vi "Find Program Files.vi"() -> (2 "filenames":string[](array[string]), 3 "Array":string[](array[string]))   [LabVIEW 2025]
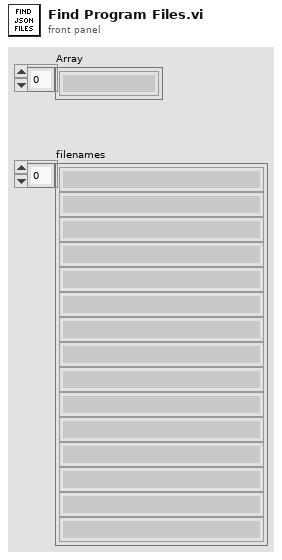
[diagram p1: front panel]
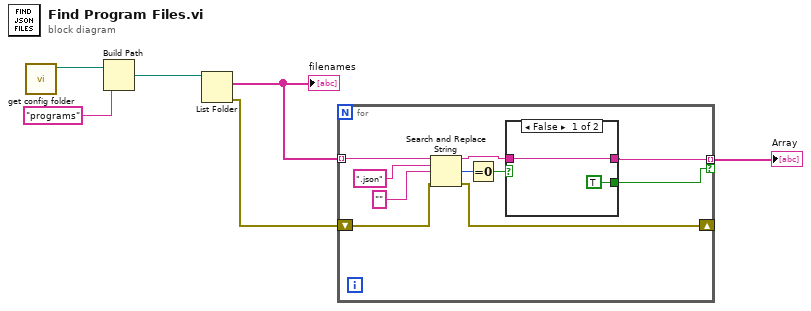
[diagram p0: block diagram]
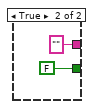
[diagram p2: hidden frame]
diagram:
  n1 = call "get config folder.vi"() -> ("Config folder path"=w1:path)  [unwired: 11 in]
  n2 = Build Path(base path=w1, name or relative path="programs") -> (appended path=w3:path)
  n3 = List Folder(path=w3) -> (filenames=w4:string[], error out=w5:errorcluster)  [unwired: 3 in, 2 out]
  "filenames" <- w4
  n4 = for {
    tunnel: w4 -> [w16] mode=indexing
    shift-right: [w11] -> _
    shift-left: w5 -> [w12]
    tunnel: [w8] -> w6 mode=indexing if=w7
    n5 = Search and Replace String(input string=w16, search string=".json", replace string="" ("replace string (\"\")"), error in=w12) -> (result string=w9:string, number of replacements=w14:i32, error out=w11:errorcluster)  [unwired: 4 in, 1 out]
    n6 = Equal To 0?(x=w14) -> (x = 0?=w10:bool)
    n7 = case shown="False" w10 {
      tunnel: w9 -> [w18 _]
      tunnel: [w18 "" ("result string")] -> w8
      tunnel: [TRUE FALSE] -> w7
      frame False {
      }
      frame True {
      }
    }
  }
  "Array" <- w6
